vi "Measurement Logic.vi"() -> ()   [LabVIEW 2024, in "Eff And Load Reg_Channel Ganging.lvlib"]
uses:
  Eff And Load Reg_Channel Ganging.lvlib
  Measurement Configuration.ctl
  Measurement Results.ctl
  <vilib>/Plug-In SDKs/Measurements/Measure Call Context/Measure Call Context.lvclass
  <instrlib>/niDCPower/nidcpower.llb/niDCPower Source Mode.ctl
  <instrlib>/niDCPower/nidcpower.llb/niDCPower Output Function.ctl
  <instrlib>/niDCPower/nidcpower.llb/niDCPower Wait For Event - Event.ctl
  shared subVIs/Triggers and Events/NIDCPower_channel_ganging - Configure Digital Edge Source Trigger.vi
  shared subVIs/Triggers and Events/NIDCPower_channel_ganging - Configure Digital Edge Measure Trigger.vi
  <vilib>/Plug-In SDKs/Measurements/Measure Call Context/Accessor/Is Canceled.vi
panel:
  out "measure call context out":refnum<class "Measure Call Context.lvclass">
  in  "measure call context in":refnum<class "Measure Call Context.lvclass">
  out "measurement results":T1
  in  "measurement configuration":T2={"Source master resource name"="", "Source slave resource names"=[], "Load master resource name"="", "Load slave resource names"=[], "Source system configuration"=enum."Parallel", "Source start voltage"=6.0, "Source stop voltage"=14.0, "Source voltage sweep points"=4, "Source voltage level range"=20.0, "Source sense"=1009, "Source limit symmetry"=enum."Asymmetric", "Source current limit range"=25.0, "Source current limit low"=-0.6, "Source current limit high"=25.0, "Source transient response"=1038, "Source voltage gain bandwidth"=2000.0, "Source voltage compensation frequency"=3530.0, "Source voltage pole-zero ratio"=2.0, "Load system configuration"=enum."Parallel", "Load start current"=1.0, "Load stop current"=50.0, "Load current sweep points/points per decade"=10, "Load sweep type"="Logarithmic", "Load current level range"=80.0, "Load sense"=1009, "Load limit symmetry"=enum."Symmetric", "Load voltage limit range"=6.0, "Load voltage limit low"=0.0, "Load voltage limit high"=inf, "Load transient response"=1038, "Load current gain bandwidth"=14000.0, "Load current compensation frequency"=180000.0, "Load current pole-zero ratio"=0.3, "DUT setup time"=1.0, "Source delay"=0.005, "Aperture time"=0.005, "Nominal output voltage"=1.0, "Mode of operation"=enum."Power on the DUT", "Measurement timeout"=0.0} {"Source start voltage" format="%#_6p"; "Load sense" items=["Local"=1008, "Remote"=1009]; "Load transient response" items=["Slow"=1041, "Normal"=1038, "Fast"=1039, "Custom"=1042]; "Source sense" items=["Local"=1008, "Remote"=1009]; "Source transient response" items=["Slow"=1041, "Normal"=1038, "Fast"=1039, "Custom"=1042]; "Load voltage limit high" format="%#_6p"; "Load voltage limit low" format="%#_6p"; "Load voltage limit range" format="%#_6p"; "Source current limit high" format="%#_6p"; "Source current limit low" format="%#_6p"; "Source current limit range" format="%#_6p"; "Source voltage level range" format="%#_6p"}
  out "error out":errorcluster
  in  "error in":errorcluster
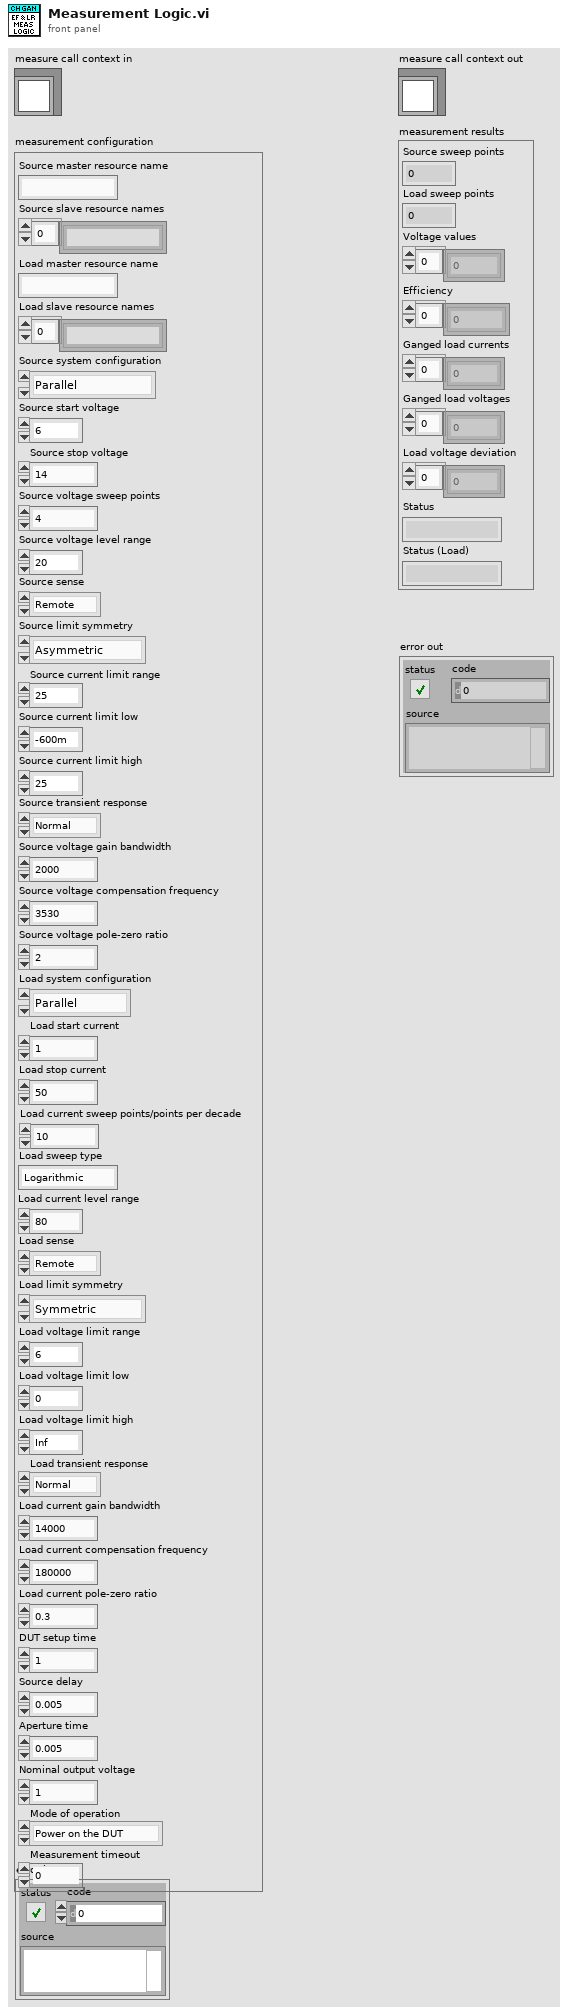
[diagram p1: front panel]
types:
  T1 = typedef "Eff And Load Reg_Channel Ganging.lvlib/Measurement Results.ctl" = cluster{"Source sweep points":i32, "Load sweep points":i32, "Voltage values":dbl[], "Efficiency":dbl[], "Ganged load currents":dbl[], "Ganged load voltages":dbl[], "Load voltage deviation":dbl[], "Status":string, "Status (Load)":string}
  T2 = typedef "Eff And Load Reg_Channel Ganging.lvlib/Measurement Configuration.ctl" = cluster{"Source master resource name":string, "Source slave resource names":string[], "Load master resource name":string, "Load slave resource names":string[], "Source system configuration":enum32{"Series", "Parallel", "Manual"}, "Source start voltage":dbl, "Source stop voltage":dbl, "Source voltage sweep points":i32, "Source voltage level range":dbl, "Source sense":i32, "Source limit symmetry":enum32{"Symmetric", "Asymmetric"}, "Source current limit range":dbl, "Source current limit low":dbl, "Source current limit high":dbl, "Source transient response":i32, "Source voltage gain bandwidth":dbl, "Source voltage compensation frequency":dbl, "Source voltage pole-zero ratio":dbl, "Load system configuration":enum32{"Series", "Parallel", "Manual"}, "Load start current":dbl, "Load stop current":dbl, "Load current sweep points/points per decade":i32, "Load sweep type":string, "Load current level range":dbl, "Load sense":i32, "Load limit symmetry":enum32{"Symmetric", "Asymmetric"}, "Load voltage limit range":dbl, "Load voltage limit low":dbl, "Load voltage limit high":dbl, "Load transient response":i32, "Load current gain bandwidth":dbl, "Load current compensation frequency":dbl, "Load current pole-zero ratio":dbl, "DUT setup time":dbl, "Source delay":dbl, "Aperture time":dbl, "Nominal output voltage":dbl, "Mode of operation":enum32{"Power on the DUT", "Perform measurement", "Power off the DUT"}, "Measurement timeout":dbl}
  T3 = enum32{"Power on the DUT", "Perform measurement", "Power off the DUT"}
  T4 = typedef "niDCPower Output Function.ctl" = i32
  T5 = typedef "niDCPower Source Mode.ctl" = i32
  T6 = typedef "NIDCPower_channel_ganging - ctl - channel def.ctl" = cluster{"resource name":refnum<k15>, "channels":string, "Channel Mode":T7}
  T7 = typedef "NIDCPower_channel_ganging - ctl - channel mode.ctl" = enum32{"Master", "Slave", "Slave - Inverted"}
  T8 = typedef "NIDCPower_channel_ganging - ctl - ganged session.ctl" = cluster{"Ganged Config":T9, "Session List":refnum<k15>[], "Session Mode":T7[], "Channel":string[]}
  T9 = typedef "NIDCPower_channel_ganging - ctl - ganged config.ctl" = enum32{"Series", "Parallel", "Manual"}
  T10 = typedef "niDCPower Wait For Event - Event.ctl" = i32
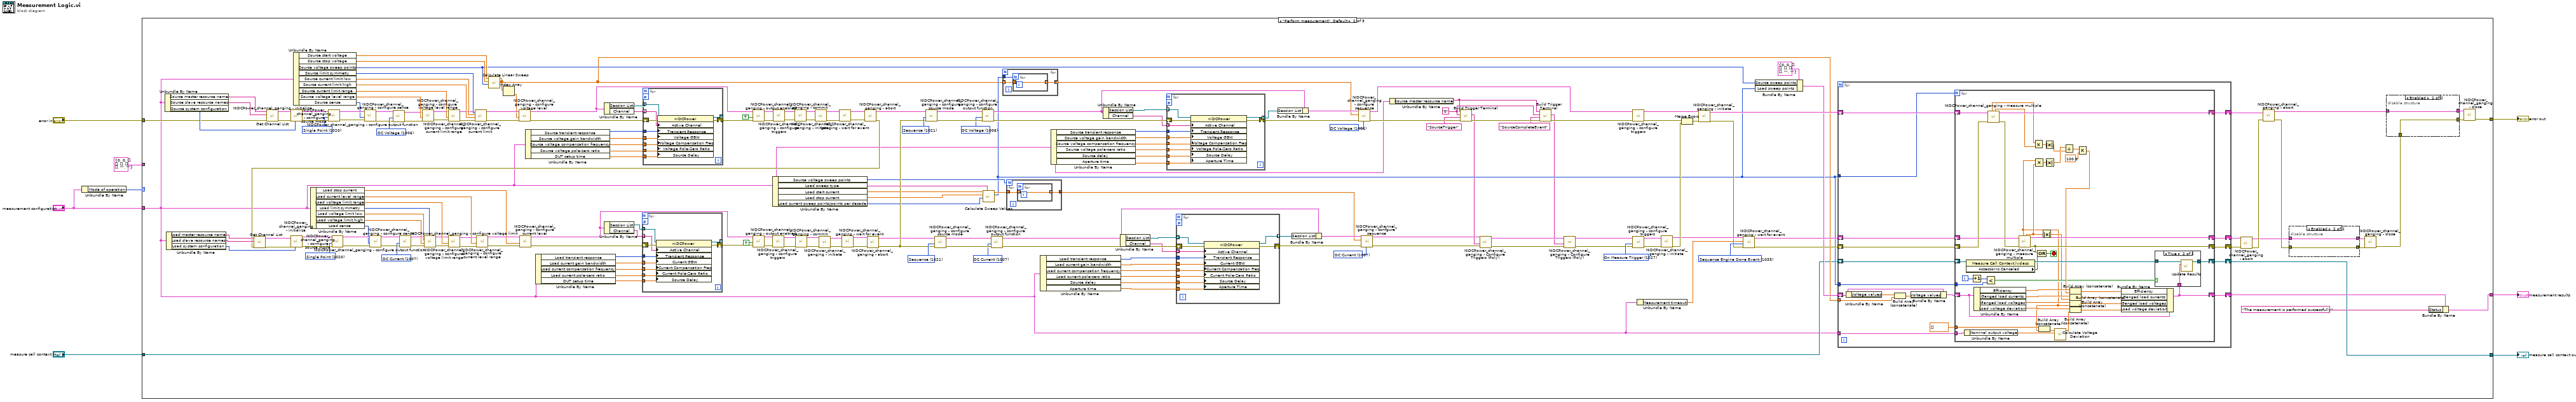
[diagram p0: block diagram]
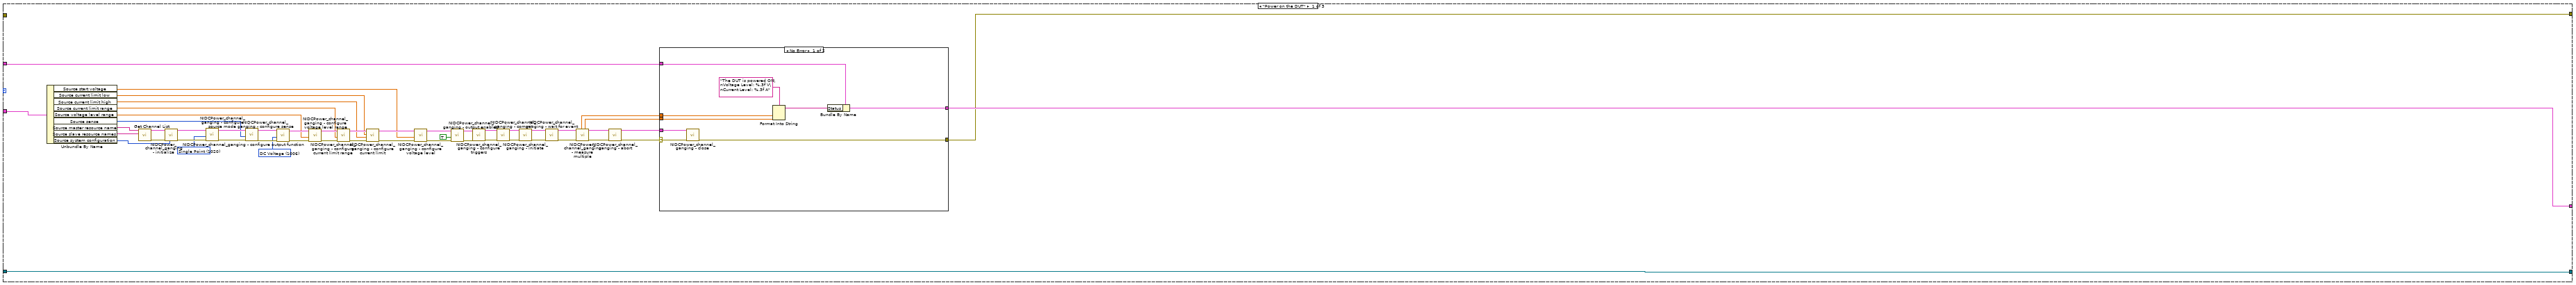
[diagram p2: hidden frame]
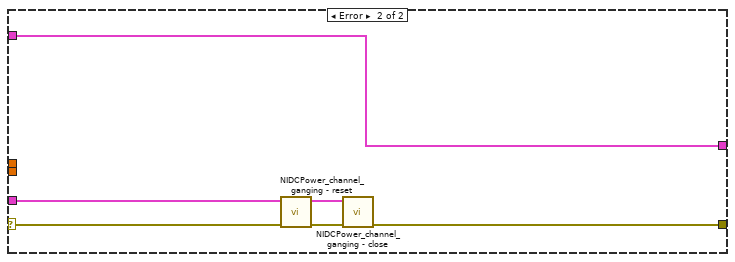
[diagram p3: hidden frame]
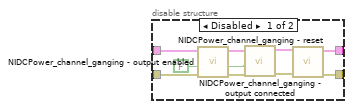
[diagram p4: hidden frame]
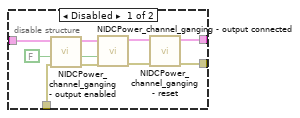
[diagram p5: hidden frame]
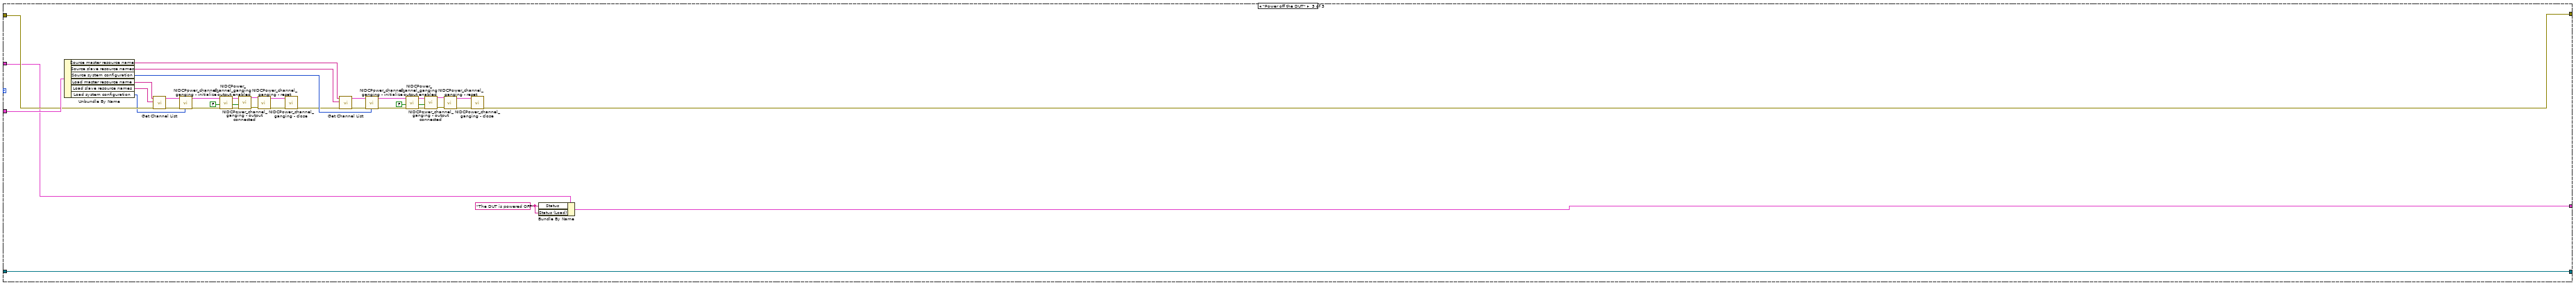
[diagram p7: hidden frame]
diagram:
  n1 = Unbundle By Name("measurement configuration") -> ("Mode of operation"=w3:T3)
  n2 = case shown="\"Perform measurement\", Default" w3 {
    tunnel: [w12 w78 w416] -> w8
    tunnel: [w10 w139 w415] -> w7
    tunnel: [w11 w138 w417] -> w6
    tunnel: "measurement configuration" -> [w14 w76 w448]
    tunnel: "measure call context in" -> [w10 w81 w415]
    tunnel: "error in" -> [_ w80 w442]
    tunnel: T1 {"Source sweep points"=0, "Load sweep points"=0, "Voltage values"=[], "Efficiency"=[], "Ganged load currents"=[], "Ganged load voltages"=[], "Load voltage deviation"=[], "Status"="", "Status (Load)"=""} ("measurement results") -> [w13 _ w418]
    frame "Power on the DUT" {
      w39 = T4 1006 items=["DC Voltage"=1006, "DC Current"=1007, "Pulse Voltage"=1049, "Pulse Current"=1050] ("output function")
      w43 = T5 1020 items=["Single Point"=1020, "Sequence"=1021] ("source mode")
      n3 = Unbundle By Name(w14) -> ("Source start voltage"=w34:dbl, "Source current limit low"=w36:dbl, "Source current limit high"=w35:dbl, "Source current limit range"=w37:dbl, "Source voltage level range"=w38:dbl, "Source sense"=w40:i32, "Source master resource name"=w42:string, "Source slave resource names"=w41:string[], "Source system configuration"=w9:enum32{"Series", "Parallel", "Manual"})
      n4 = call "Get Channel List.vi"("Slave resource names"=w41, "Master resouce name"=w42) -> ("error out"=w44:errorcluster, "Channel List"=w45:T6[])  [unwired: 8 in]
      n5 = call "NIDCPower_channel_ganging - initialize.vi"("Ganged Config"=w9, "error in (no error)"=w44, "Channel List"=w45) -> ("error out"=w58:errorcluster, "Ganged Session Out"=w59:T8)  [unwired: 7 in]
      n6 = call "NIDCPower_channel_ganging - configure source mode.vi"("error in (no error)"=w58, "source mode"=w43, "Ganged Session In"=w59) -> ("error out"=w50:errorcluster, "Ganged Session Out"=w51:T8)  [unwired: 7 in]
      n7 = call "NIDCPower_channel_ganging - configure sense.vi"("error in (no error)"=w50, "sense"=w40, "Ganged Session In"=w51) -> ("error out"=w48:errorcluster, "Ganged Session Out"=w49:T8)  [unwired: 7 in]
      n8 = call "NIDCPower_channel_ganging - configure output function.vi"("error in (no error)"=w48, "output function"=w39, "Ganged Session In"=w49) -> ("error out"=w46:errorcluster, "Ganged Session Out"=w47:T8)  [unwired: 7 in]
      n9 = call "NIDCPower_channel_ganging - configure voltage level range.vi"("error in (no error)"=w46, "voltage level range"=w38, "Ganged Session In"=w47) -> ("error out"=w54:errorcluster, "Ganged Session Out"=w57:T8)  [unwired: 7 in]
      n10 = call "NIDCPower_channel_ganging - configure current limit range.vi"("error in (no error)"=w54, "current limit range"=w37, "Ganged Session In"=w57) -> ("error out"=w53:errorcluster, "Ganged Session Out"=w56:T8)  [unwired: 7 in]
      n11 = call "NIDCPower_channel_ganging - configure current limit.vi"("error in (no error)"=w53, "Current limit/hi"=w35, "Current limit lo"=w36, "Ganged Session In"=w56) -> ("error out"=w52:errorcluster, "Ganged Session Out"=w55:T8)  [unwired: 6 in]
      n12 = call "NIDCPower_channel_ganging - configure voltage level.vi"("error in (no error)"=w52, "voltage level"=w34, "Ganged Session In"=w55) -> ("error out"=w23:errorcluster, "Ganged Session Out"=w24:T8)  [unwired: 7 in]
      n13 = call "NIDCPower_channel_ganging - output enabled.vi"("error in (no error)"=w23, "output enabled"=TRUE, "Ganged Session In"=w24) -> ("error out"=w31:errorcluster, "Ganged Session Out"=w30:T8)  [unwired: 7 in]
      n14 = call "NIDCPower_channel_ganging - configure triggers.vi"("error in (no error)"=w31, "Ganged Session In"=w30) -> ("error out"=w33:errorcluster, "Ganged Session Out"=w32:T8)  [unwired: 8 in]
      n15 = call "NIDCPower_channel_ganging - commit.vi"("error in (no error)"=w33, "Ganged Session In"=w32) -> ("error out"=w28:errorcluster, "Ganged Session Out"=w29:T8)  [unwired: 8 in]
      n16 = call "NIDCPower_channel_ganging - initiate.vi"("error in (no error)"=w28, "Ganged Session In"=w29) -> ("error out"=w26:errorcluster, "Ganged Session Out"=w27:T8)  [unwired: 8 in]
      n17 = call "NIDCPower_channel_ganging - wait for event.vi"("error in (no error)"=w26, "Ganged Session in"=w27) -> ("error out"=w21:errorcluster, "Ganged Session Out"=w22:T8)  [unwired: 8 in]
      n18 = call "NIDCPower_channel_ganging - measure multiple.vi"("error in (no error)"=w21, "Ganged Session In"=w22) -> ("error out"=w19:errorcluster, "Ganged Session Out"=w20:T8, "ganged current measurement"=w15:dbl, "ganged voltage measurement"=w16:dbl)  [unwired: 2 in, 4 out]
      n19 = call "NIDCPower_channel_ganging - abort.vi"("error in (no error)"=w19, "Ganged Session In"=w20) -> ("error out"=w18:errorcluster, "Ganged Session Out"=w17:T8)  [unwired: 8 in]
      n20 = case shown="No Error" w18 {
        selector: w18 -> [w67 w72]
        tunnel: w17 -> [w68 w74]
        tunnel: w16 -> [w66 _]
        tunnel: w15 -> [w65 _]
        tunnel: w13 -> [w63 w70]
        tunnel: [w61 w69] -> w11
        tunnel: [w60 w70] -> w12
        frame No Error {
          n21 = call "NIDCPower_channel_ganging - close.vi"("error in (no error)"=w67, "Ganged Session In"=w68) -> ("error out"=w61:errorcluster)  [unwired: 9 in]
          n22 = Format Into String(format string="The DUT is powered ON\nVoltage Level: %.3f V\nCurrent Level: %.3f A", w66, w65) -> (resulting string=w62:string)  [unwired: 2 in, 1 out]
          n23 = Bundle By Name(cluster=w63, "Status"=w62) -> (w60:T1)
        }
        frame Error {
          n24 = call "NIDCPower_channel_ganging - reset.vi"("error in (no error)"=w72, "Ganged Session In"=w74) -> ("error out"=w71:errorcluster, "Ganged Session Out"=w73:T8)  [unwired: 8 in]
          n25 = call "NIDCPower_channel_ganging - close.vi"("error in (no error)"=w71, "Ganged Session In"=w73) -> ("error out"=w69:errorcluster)  [unwired: 9 in]
        }
      }
    }
    frame "Perform measurement", Default {
      w103 = T4 1007 items=["DC Voltage"=1006, "DC Current"=1007, "Pulse Voltage"=1049, "Pulse Current"=1050] ("output function")
      w104 = T4 1006 items=["DC Voltage"=1006, "DC Current"=1007, "Pulse Voltage"=1049, "Pulse Current"=1050] ("output function")
      w133 = "0" ("Channel Name")
      w178 = 1027 items=["Automatically after Source Complete"=1025, "On Demand"=1026, "On Measure Trigger"=1027] ("Measure When")
      w175 = T4 1006 items=["DC Voltage"=1006, "DC Current"=1007, "Pulse Voltage"=1049, "Pulse Current"=1050] ("output function")
      w180 = T5 1021 items=["Single Point"=1020, "Sequence"=1021] ("source mode")
      w181 = T5 1021 items=["Single Point"=1020, "Sequence"=1021] ("source mode")
      w112 = T4 1007 items=["DC Voltage"=1006, "DC Current"=1007, "Pulse Voltage"=1049, "Pulse Current"=1050] ("output function")
      w228 = T10 1033 items=["Source Complete Event"=1030, "Measure Complete Event"=1031, "Sequence Iteration Complete Event"=1032, "Sequence Engine Done Event"=1033, "Pulse Complete Event"=1051, "Ready For Pulse Trigger Event"=1052] ("event")
      w229 = T4 1007 items=["DC Voltage"=1006, "DC Current"=1007, "Pulse Voltage"=1049, "Pulse Current"=1050] ("output function")
      w242 = T4 1006 items=["DC Voltage"=1006, "DC Current"=1007, "Pulse Voltage"=1049, "Pulse Current"=1050] ("output function")
      w274 = T5 1020 items=["Single Point"=1020, "Sequence"=1021] ("source mode")
      w275 = T5 1020 items=["Single Point"=1020, "Sequence"=1021] ("source mode")
      n26 = Unbundle By Name(w76) -> ("Source master resource name"=w124:string, "Source slave resource names"=w123:string[], "Source system configuration"=w253:enum32{"Series", "Parallel", "Manual"})
      n27 = Unbundle By Name(w76) -> ("Load master resource name"=w120:string, "Load slave resource names"=w119:string[], "Load system configuration"=w252:enum32{"Series", "Parallel", "Manual"})
      n28 = call "Get Channel List.vi"("error in (no error)"=w80, "Slave resource names"=w123, "Master resouce name"=w124) -> ("error out"=w125:errorcluster, "Channel List"=w126:T6[])  [unwired: 7 in]
      n29 = call "NIDCPower_channel_ganging - initialize.vi"("Ganged Config"=w253, "error in (no error)"=w125, "Channel List"=w126) -> ("error out"=w276:errorcluster, "Ganged Session Out"=w277:T8)  [unwired: 7 in]
      n30 = Unbundle By Name(w76) -> ("Source start voltage"=w155:dbl, "Source stop voltage"=w154:dbl, "Source voltage sweep points"=w142:i32, "Source limit symmetry"=w259:enum32{"Symmetric", "Asymmetric"}, "Source current limit low"=w260:dbl, "Source current limit high"=w261:dbl, "Source current limit range"=w262:dbl, "Source voltage level range"=w263:dbl, "Source sense"=w130:i32)
      n31 = Unbundle By Name(w76) -> ("Load stop current"=w144:dbl, "Load current level range"=w254:dbl, "Load voltage limit range"=w255:dbl, "Load limit symmetry"=w258:enum32{"Symmetric", "Asymmetric"}, "Load voltage limit low"=w257:dbl, "Load voltage limit high"=w256:dbl, "Load sense"=w131:i32)
      n32 = call "NIDCPower_channel_ganging - configure source mode.vi"("error in (no error)"=w276, "source mode"=w275, "Ganged Session In"=w277) -> ("error out"=w225:errorcluster, "Ganged Session Out"=w226:T8)  [unwired: 7 in]
      n33 = call "NIDCPower_channel_ganging - configure sense.vi"("error in (no error)"=w225, "sense"=w130, "Ganged Session In"=w226) -> ("error out"=w223:errorcluster, "Ganged Session Out"=w224:T8)  [unwired: 7 in]
      n34 = call "NIDCPower_channel_ganging - configure output function.vi"("error in (no error)"=w223, "output function"=w242, "Ganged Session In"=w224) -> ("error out"=w221:errorcluster, "Ganged Session Out"=w222:T8)  [unwired: 7 in]
      n35 = call "NIDCPower_channel_ganging - configure voltage level range.vi"("error in (no error)"=w221, "voltage level range"=w263, "Ganged Session In"=w222) -> ("error out"=w238:errorcluster, "Ganged Session Out"=w241:T8)  [unwired: 7 in]
      n36 = call "NIDCPower_channel_ganging - configure current limit range.vi"("error in (no error)"=w238, "current limit range"=w262, "Ganged Session In"=w241) -> ("error out"=w237:errorcluster, "Ganged Session Out"=w240:T8)  [unwired: 7 in]
      n37 = call "NIDCPower_channel_ganging - configure current limit.vi"("Limit Symmetry"=w259, "error in (no error)"=w237, "Current limit/hi"=w261, "Current limit lo"=w260, "Ganged Session In"=w240) -> ("error out"=w236:errorcluster, "Ganged Session Out"=w239:T8)  [unwired: 5 in]
      n38 = call "Calculate Linear Sweep.vi"("Points"=w142, "Stop level"=w154, "Start level"=w155) -> ("Values"=w132:dbl[])  [unwired: 8 in]
      n39 = Index Array(array=w132) -> (element=w156:dbl)  [unwired: 1 in]
      n40 = call "NIDCPower_channel_ganging - configure voltage level.vi"("error in (no error)"=w236, "voltage level"=w156, "Ganged Session In"=w239) -> ("error out"=w196:errorcluster, "Ganged Session Out"=w190:T8)  [unwired: 7 in]
      n41 = Unbundle By Name(w76) -> ("Source transient response"=w97:i32, "Source voltage gain bandwidth"=w93:dbl, "Source voltage compensation frequency"=w92:dbl, "Source voltage pole-zero ratio"=w91:dbl, "DUT setup time"=w94:dbl)
      n42 = Unbundle By Name(w76) -> ("Load transient response"=w96:i32, "Load current gain bandwidth"=w90:dbl, "Load current compensation frequency"=w89:dbl, "Load current pole-zero ratio"=w88:dbl, "DUT setup time"=w95:dbl)
      n43 = Unbundle By Name(w190) -> ("Session List"=w194:refnum<k15>[], "Channel"=w193:string[])
      n44 = for {
        tunnel: [w337] -> _ mode=indexing
        shift-right: [w335] -> w195
        shift-left: w196 -> [w336]
        workers-P: _ -> [_]
        tunnel: w194 -> [w334] mode=indexing
        tunnel: w193 -> [w333] mode=indexing
        tunnel: w97 -> [w332]
        tunnel: w94 -> [w331]
        tunnel: w93 -> [w330]
        tunnel: w92 -> [w329]
        tunnel: w91 -> [w328]
        n45 = property class="niDCPower"(reference=w334, error in=w336, "Active Channel"=w333, "Transient Response"=w332, "Voltage GBW"=w330, "Voltage Compensation Freq"=w329, "Voltage Pole-Zero Ratio"=w328, "Source Delay"=w331) -> (reference out=w337:refnum<k15>, error out=w335:errorcluster)
      }
      n46 = call "NIDCPower_channel_ganging - output enabled.vi"("error in (no error)"=w195, "output enabled"=TRUE, "Ganged Session In"=w190) -> ("error out"=w199:errorcluster, "Ganged Session Out"=w200:T8)  [unwired: 7 in]
      n47 = Unbundle By Name(w76) -> ("Source voltage sweep points"=w145:i32, "Load sweep type"=w129:string, "Load start current"=w153:dbl, "Load stop current"=w152:dbl, "Load current sweep points/points per decade"=w151:i32)
      n48 = call "NIDCPower_channel_ganging - configure triggers.vi"("error in (no error)"=w199, "Ganged Session In"=w200) -> ("error out"=w197:errorcluster, "Ganged Session Out"=w198:T8)  [unwired: 8 in]
      n49 = call "NIDCPower_channel_ganging - commit.vi"("error in (no error)"=w197, "Ganged Session In"=w198) -> ("error out"=w206:errorcluster, "Ganged Session Out"=w205:T8)  [unwired: 8 in]
      n50 = call "NIDCPower_channel_ganging - initiate.vi"("error in (no error)"=w206, "Ganged Session In"=w205) -> ("error out"=w208:errorcluster, "Ganged Session Out"=w207:T8)  [unwired: 8 in]
      n51 = call "NIDCPower_channel_ganging - wait for event.vi"("error in (no error)"=w208, "Ganged Session in"=w207) -> ("error out"=w210:errorcluster, "Ganged Session Out"=w209:T8)  [unwired: 8 in]
      n52 = call "NIDCPower_channel_ganging - abort.vi"("error in (no error)"=w210, "Ganged Session In"=w209) -> ("error out"=w118:errorcluster, "Ganged Session Out"=w179:T8)  [unwired: 8 in]
      n53 = call "Get Channel List.vi"("error in (no error)"=w118, "Slave resource names"=w119, "Master resouce name"=w120) -> ("error out"=w122:errorcluster, "Channel List"=w121:T6[])  [unwired: 7 in]
      n54 = call "NIDCPower_channel_ganging - initialize.vi"("Ganged Config"=w252, "error in (no error)"=w122, "Channel List"=w121) -> ("error out"=w273:errorcluster, "Ganged Session Out"=w272:T8)  [unwired: 7 in]
      n55 = call "NIDCPower_channel_ganging - configure source mode.vi"("error in (no error)"=w273, "source mode"=w274, "Ganged Session In"=w272) -> ("error out"=w219:errorcluster, "Ganged Session Out"=w220:T8)  [unwired: 7 in]
      n56 = call "NIDCPower_channel_ganging - configure sense.vi"("error in (no error)"=w219, "sense"=w131, "Ganged Session In"=w220) -> ("error out"=w217:errorcluster, "Ganged Session Out"=w218:T8)  [unwired: 7 in]
      n57 = call "NIDCPower_channel_ganging - configure output function.vi"("error in (no error)"=w217, "output function"=w229, "Ganged Session In"=w218) -> ("error out"=w270:errorcluster, "Ganged Session Out"=w271:T8)  [unwired: 7 in]
      n58 = call "NIDCPower_channel_ganging - configure voltage limit.vi"("Limit Symmetry"=w258, "error in (no error)"=w270, "voltage limit/hi"=w256, "voltage limit lo"=w257, "Ganged Session In"=w271) -> ("error out"=w234:errorcluster, "Ganged Session Out"=w235:T8)  [unwired: 5 in]
      n59 = call "NIDCPower_channel_ganging - configure voltage limit range.vi"("error in (no error)"=w234, "voltage level range"=w255, "Ganged Session In"=w235) -> ("error out"=w232:errorcluster, "Ganged Session Out"=w233:T8)  [unwired: 7 in]
      n60 = call "NIDCPower_channel_ganging - configure current level range.vi"("error in (no error)"=w232, "current level range"=w254, "Ganged Session In"=w233) -> ("error out"=w230:errorcluster, "Ganged Session Out"=w231:T8)  [unwired: 7 in]
      n61 = call "NIDCPower_channel_ganging - configure current level.vi"("error in (no error)"=w230, "current level"=w144, "Ganged Session In"=w231) -> ("error out"=w192:errorcluster, "Ganged Session Out"=w189:T8)  [unwired: 7 in]
      n62 = Unbundle By Name(w189) -> ("Session List"=w188:refnum<k15>[], "Channel"=w187:string[])
      n63 = for {
        tunnel: [w327] -> _ mode=indexing
        shift-right: [w325] -> w191
        shift-left: w192 -> [w326]
        workers-P: _ -> [_]
        tunnel: w188 -> [w324] mode=indexing
        tunnel: w187 -> [w323] mode=indexing
        tunnel: w96 -> [w322]
        tunnel: w95 -> [w321]
        tunnel: w90 -> [w320]
        tunnel: w89 -> [w319]
        tunnel: w88 -> [w318]
        n64 = property class="niDCPower"(reference=w324, error in=w326, "Active Channel"=w323, "Transient Response"=w322, "Current GBW"=w320, "Current Compensation Freq"=w319, "Current Pole-Zero Ratio"=w318, "Source Delay"=w321) -> (reference out=w327:refnum<k15>, error out=w325:errorcluster)
      }
      n65 = call "NIDCPower_channel_ganging - output enabled.vi"("error in (no error)"=w191, "output enabled"=TRUE, "Ganged Session In"=w189) -> ("error out"=w203:errorcluster, "Ganged Session Out"=w204:T8)  [unwired: 7 in]
      n66 = call "NIDCPower_channel_ganging - configure triggers.vi"("error in (no error)"=w203, "Ganged Session In"=w204) -> ("error out"=w201:errorcluster, "Ganged Session Out"=w202:T8)  [unwired: 8 in]
      n67 = call "NIDCPower_channel_ganging - commit.vi"("error in (no error)"=w201, "Ganged Session In"=w202) -> ("error out"=w215:errorcluster, "Ganged Session Out"=w216:T8)  [unwired: 8 in]
      n68 = call "NIDCPower_channel_ganging - initiate.vi"("error in (no error)"=w215, "Ganged Session In"=w216) -> ("error out"=w213:errorcluster, "Ganged Session Out"=w214:T8)  [unwired: 8 in]
      n69 = call "NIDCPower_channel_ganging - wait for event.vi"("error in (no error)"=w213, "Ganged Session in"=w214) -> ("error out"=w211:errorcluster, "Ganged Session Out"=w212:T8)  [unwired: 8 in]
      n70 = call "NIDCPower_channel_ganging - abort.vi"("error in (no error)"=w211, "Ganged Session In"=w212) -> ("error out"=w157:errorcluster, "Ganged Session Out"=w182:T8)  [unwired: 8 in]
      n71 = call "NIDCPower_channel_ganging - configure source mode.vi"("error in (no error)"=w157, "source mode"=w180, "Ganged Session In"=w179) -> ("error out"=w183:errorcluster, "Ganged Session Out"=w184:T8)  [unwired: 7 in]
      n72 = call "NIDCPower_channel_ganging - configure source mode.vi"("error in (no error)"=w157, "source mode"=w181, "Ganged Session In"=w182) -> ("error out"=w186:errorcluster, "Ganged Session Out"=w185:T8)  [unwired: 7 in]
      n73 = call "NIDCPower_channel_ganging - configure output function.vi"("error in (no error)"=w183, "output function"=w175, "Ganged Session In"=w184) -> ("error out"=w176:errorcluster, "Ganged Session Out"=w177:T8)  [unwired: 7 in]
      n74 = call "Calculate Sweep Values.vi"("Sweep type"=w129, "Points"=w151, "Stop level"=w152, "Start level"=w153) -> ("Sweep points"=w141:i32, "Sweep values"=w150:dbl[])  [unwired: 5 in, 1 out]
      n75 = call "NIDCPower_channel_ganging - configure output function.vi"("error in (no error)"=w186, "output function"=w112, "Ganged Session In"=w185) -> ("error out"=w162:errorcluster, "Ganged Session Out"=w163:T8)  [unwired: 7 in]
      n76 = for {
        tunnel: w132 -> [w302] mode=indexing
        tunnel: [w301] -> w109 mode=concatenating
        tunnel: w141 -> [w300]
        n77 = for {
          N: w300 -> [_]
          tunnel: w302 -> [w303]
          tunnel: [w303] -> w301 mode=indexing
        }
      }
      n78 = for {
        N: w145 -> [_]
        tunnel: w150 -> [w305]
        tunnel: [w304] -> w113 mode=concatenating
        n79 = for {
          tunnel: w305 -> [w306] mode=indexing
          tunnel: [w306] -> w304 mode=indexing
        }
      }
      n80 = Unbundle By Name(w76) -> ("Load transient response"=w102:i32, "Load current gain bandwidth"=w84:dbl, "Load current compensation frequency"=w83:dbl, "Load current pole-zero ratio"=w82:dbl, "Source delay"=w101:dbl, "Aperture time"=w100:dbl)
      n81 = Unbundle By Name(w76) -> ("Source transient response"=w105:i32, "Source voltage gain bandwidth"=w87:dbl, "Source voltage compensation frequency"=w86:dbl, "Source voltage pole-zero ratio"=w85:dbl, "Source delay"=w99:dbl, "Aperture time"=w98:dbl)
      n82 = Unbundle By Name(w177) -> ("Session List"=w267:refnum<k15>[], "Channel"=w161:string[])
      n83 = Unbundle By Name(w163) -> ("Session List"=w160:refnum<k15>[], "Channel"=w159:string[])
      n84 = for {
        tunnel: [w348] -> w266 mode=indexing
        shift-right: [w346] -> w108
        shift-left: w176 -> [w347]
        workers-P: _ -> [_]
        tunnel: w267 -> [w345] mode=indexing
        tunnel: w161 -> [w344] mode=indexing
        tunnel: w105 -> [w343]
        tunnel: w99 -> [w342]
        tunnel: w98 -> [w341]
        tunnel: w87 -> [w340]
        tunnel: w86 -> [w339]
        tunnel: w85 -> [w338]
        n85 = property class="niDCPower"(reference=w345, error in=w347, "Active Channel"=w344, "Transient Response"=w343, "Voltage GBW"=w340, "Voltage Compensation Freq"=w339, "Voltage Pole-Zero Ratio"=w338, "Source Delay"=w342, "Aperture Time"=w341) -> (reference out=w348:refnum<k15>, error out=w346:errorcluster)
      }
      n86 = for {
        tunnel: [w317] -> w158 mode=indexing
        shift-right: [w315] -> w116
        shift-left: w162 -> [w316]
        workers-P: _ -> [_]
        tunnel: w160 -> [w314] mode=indexing
        tunnel: w159 -> [w313] mode=indexing
        tunnel: w102 -> [w312]
        tunnel: w101 -> [w311]
        tunnel: w100 -> [w310]
        tunnel: w84 -> [w309]
        tunnel: w83 -> [w308]
        tunnel: w82 -> [w307]
        n87 = property class="niDCPower"(reference=w314, error in=w316, "Active Channel"=w313, "Transient Response"=w312, "Current GBW"=w309, "Current Compensation Freq"=w308, "Current Pole-Zero Ratio"=w307, "Source Delay"=w311, "Aperture Time"=w310) -> (reference out=w317:refnum<k15>, error out=w315:errorcluster)
      }
      n88 = Bundle By Name(cluster=w177, "Session List"=w266) -> (w111:T8)
      n89 = Bundle By Name(cluster=w163, "Session List"=w158) -> (w117:T8)
      n90 = call "NIDCPower_channel_ganging - confgure sequence.vi"("output function"=w104, "error in (no error)"=w108, "Values"=w109, "Ganged Session In"=w111) -> ("error out"=w107:errorcluster, "Ganged Session Out"=w110:T8)  [unwired: 6 in]
      n91 = call "NIDCPower_channel_ganging - confgure sequence.vi"("output function"=w103, "error in (no error)"=w116, "Values"=w113, "Ganged Session In"=w117) -> ("error out"=w114:errorcluster, "Ganged Session Out"=w115:T8)  [unwired: 6 in]
      n92 = Unbundle By Name(w76) -> ("Source master resource name"=w106:string)
      n93 = call "Build Trigger Terminal.vi"("error in (no error)"=w107, "Trigger/Event Name"="SourceTrigger", "Channel Name"=w133, "Resource Name"=w106) -> ("error out"=w149:errorcluster, "Terminal Name"=w128:string)  [unwired: 6 in]
      n94 = call-poly "NIDCPower_channel_ganging - Configure Triggers (Poly).vi"("error in (no error)"=w114, "output terminal"=w128, "Ganged Session in"=w115) -> ("error out"=w134:errorcluster, "Ganged Session out"=w135:T8)  [unwired: 7 in]
      n95 = call "Build Trigger Terminal.vi"("error in (no error)"=w149, "Trigger/Event Name"="SourceCompleteEvent", "Channel Name"=w133, "Resource Name"=w106) -> ("error out"=w148:errorcluster, "Terminal Name"=w127:string)  [unwired: 6 in]
      n96 = call-poly "NIDCPower_channel_ganging - Configure Triggers (Poly).vi"("error in (no error)"=w134, "output terminal"=w127, "Ganged Session in"=w135) -> ("error out"=w136:errorcluster, "Ganged Session out"=w137:T8)  [unwired: 7 in]
      n97 = call "NIDCPower_channel_ganging - configure triggers.vi"("error in (no error)"=w148, "Ganged Session In"=w110) -> ("error out"=w244:errorcluster, "Ganged Session Out"=w245:T8)  [unwired: 8 in]
      n98 = call "NIDCPower_channel_ganging - configure triggers.vi"("error in (no error)"=w136, "Measure When"=w178, "Ganged Session In"=w137) -> ("error out"=w264:errorcluster, "Ganged Session Out"=w265:T8)  [unwired: 7 in]
      n99 = Unbundle By Name(w76) -> ("Measurement timeout"=w75:dbl)
      n100 = call "NIDCPower_channel_ganging - initiate.vi"("error in (no error)"=w264, "Ganged Session In"=w265) -> ("error out"=w243:errorcluster, "Ganged Session Out"=w227:T8)  [unwired: 8 in]
      n101 = Merge Errors(w244, w243) -> (w246:errorcluster)
      n102 = call "NIDCPower_channel_ganging - initiate.vi"("error in (no error)"=w246, "Ganged Session In"=w245) -> ("error out"=w174:errorcluster, "Ganged Session Out"=w165:T8)  [unwired: 8 in]
      n103 = call "NIDCPower_channel_ganging - wait for event.vi"("error in (no error)"=w174, "event"=w228, "timeout (10.0)"=w75, "Ganged Session in"=w227) -> ("error out"=w169:errorcluster, "Ganged Session Out"=w167:T8)  [unwired: 6 in]
      n104 = Bundle By Name(cluster=T1 {"Source sweep points"=0, "Load sweep points"=0, "Voltage values"=[], "Efficiency"=[], "Ganged load currents"=[], "Ganged load voltages"=[], "Load voltage deviation"=[], "Status"="", "Status (Load)"=""} ("Measurement Results"), "Source sweep points"=w142, "Load sweep points"=w141) -> (w143:T1)
      n105 = for {
        shift-right: [w365] -> w168
        shift-left: w169 -> [w366]
        shift-right: [w363] -> w166
        shift-left: w167 -> [w364]
        shift-right: [w361] -> w164
        shift-left: w165 -> [w362]
        tunnel: w141 -> [w360]
        shift-right: [w358] -> w139
        shift-left: w81 -> [w359]
        shift-right: [w357] -> w79
        shift-left: w143 -> [w352]
        tunnel: w141 -> [w356]
        tunnel: w132 -> [w351] mode=indexing
        tunnel: w76 -> [w350]
        n106 = Unbundle By Name(w352) -> ("Voltage values"=w355:dbl[])
        n107 = Build Array (concatenate)(w355, w351) -> (w354:dbl[])
        n108 = Bundle By Name(cluster=w352, "Voltage values"=w354) -> (w353:T1)
        n109 = for {
          N: w360 -> [_]
          shift-right: [w398] -> w365
          shift-left: w366 -> [w407]
          shift-right: [w408] -> w363
          shift-left: w364 -> [w409]
          shift-right: [w404] -> w361
          shift-left: w362 -> [w405]
          shift-right: [w401] -> w358
          shift-left: w359 -> [w403]
          shift-right: [w389] -> w357
          shift-left: w353 -> [w370]
          tunnel: w356 -> [w385]
          tunnel: w350 -> [w368]
          tunnel: dbl[] [] ("Efficiency") -> [w373]
          i -> [w386]
          stop <- w400 stop-if-true
          n110 = Unbundle By Name(w368) -> ("Nominal output voltage"=w374:dbl)
          n111 = property class="Measure Call Context.lvclass"(reference=w403) -> (reference out=w402:refnum<class "Measure Call Context.lvclass">, "Accessor:Is Canceled"=w399:bool)  [unwired: 1 in, 1 out]
          n112 = Increment(x=w386) -> (x+1=w387:i32)
          n113 = Unbundle By Name(w370) -> ("Efficiency"=w397:dbl[], "Ganged load currents"=w392:dbl[], "Ganged load voltages"=w375:dbl[], "Load voltage deviation"=w378:dbl[])
          n114 = Less?(x=w387, y=w385) -> (x < y?=w384:bool)
          n115 = call "NIDCPower_channel_ganging - measure multiple.vi"("error in (no error)"=w407, "Ganged Session In"=w405) -> ("error out"=w406:errorcluster, "Ganged Session Out"=w404:T8, "ganged current measurement"=w382:dbl, "ganged voltage measurement"=w381:dbl)  [unwired: 2 in, 4 out]
          n116 = call "NIDCPower_channel_ganging - measure multiple.vi"("error in (no error)"=w406, "Ganged Session In"=w409) -> ("error out"=w398:errorcluster, "Ganged Session Out"=w408:T8, "ganged current measurement"=w383:dbl, "ganged voltage measurement"=w372:dbl)  [unwired: 2 in, 4 out]
          n117 = Multiply(x=w381, y=w382) -> (x*y=w394:dbl)
          n118 = Multiply(x=w372, y=w383) -> (x*y=w393:dbl)
          n119 = Compound Arithmetic op=OR(w398, w399) -> (w400:bool)
          n120 = Build Array (concatenate)(w373, w372) -> (w371:dbl[])
          n121 = Absolute Value(x=w383) -> (abs(x)=w367:dbl)
          n122 = Absolute Value(x=w394) -> (abs(x)=w380:dbl)
          n123 = Absolute Value(x=w393) -> (abs(x)=w379:dbl)
          n124 = call "Calculate Voltage Deviation.vi"("Nominal output voltage"=w374, "Voltage measurements"=w371) -> ("Load voltage deviation"=w377:dbl[])  [unwired: 9 in]
          n125 = Divide(x=w379, y=w380) -> (x/y=w396:dbl)
          n126 = Build Array (concatenate)(w392, w367) -> (w390:dbl[])
          n127 = Build Array (concatenate)(w375, w372) -> (w369:dbl[])
          n128 = Build Array (concatenate)(w378, w377) -> (w376:dbl[])
          n129 = Multiply(x=w396, y=100.0) -> (x*y=w388:dbl)
          n130 = Build Array (concatenate)(w397, w388) -> (w391:dbl[])
          n131 = Bundle By Name(cluster=w370, "Efficiency"=w391, "Ganged load currents"=w390, "Ganged load voltages"=w369, "Load voltage deviation"=w376) -> (w389:T1)
          n132 = case shown="True" w384 {
            tunnel: w389 -> [_ w413]
            tunnel: w402 -> [w410 w412]
            tunnel: [w410 w411] -> w401
            frame False {
            }
            frame True {
              n133 = call <vilib>:"Update Results.vi"("measurement results"=w413, "measure call context in"=w412) -> ("measure call context out"=w411:refnum<class "Measure Call Context.lvclass">)  [unwired: 8 in, 1 out]
            }
          }
        }
      }
      n134 = call "NIDCPower_channel_ganging - abort.vi"("error in (no error)"=w168, "Ganged Session In"=w166) -> ("error out"=w251:errorcluster, "Ganged Session Out"=w249:T8)  [unwired: 8 in]
      n135 = call "NIDCPower_channel_ganging - abort.vi"("error in (no error)"=w251, "Ganged Session In"=w164) -> ("error out"=w250:errorcluster, "Ganged Session Out"=w247:T8)  [unwired: 8 in]
      n136 = disable-structure shown="Enabled" {
        disable-tunnel: w250 -> [w286 w287]
        disable-tunnel: w249 -> [w283 w288]
        disable-tunnel: [w279 w288] -> w173
        disable-tunnel: [w278 w287] -> w172
        frame Disabled {
          w282 = FALSE ("output enabled")
          n137 = call "NIDCPower_channel_ganging - output enabled.vi"("error in (no error)"=w286, "output enabled"=w282, "Ganged Session In"=w283) -> ("error out"=w284:errorcluster, "Ganged Session Out"=w285:T8)  [unwired: 7 in]
          n138 = call "NIDCPower_channel_ganging - output connected.vi"("error in (no error)"=w284, "output enabled"=w282, "Ganged Session In"=w285) -> ("error out"=w281:errorcluster, "Ganged Session Out"=w280:T8)  [unwired: 7 in]
          n139 = call "NIDCPower_channel_ganging - reset.vi"("error in (no error)"=w281, "Ganged Session In"=w280) -> ("error out"=w278:errorcluster, "Ganged Session Out"=w279:T8)  [unwired: 8 in]
        }
        frame Enabled {
        }
      }
      n140 = call "NIDCPower_channel_ganging - close.vi"("error in (no error)"=w172, "Ganged Session In"=w173) -> ("error out"=w248:errorcluster)  [unwired: 9 in]
      n141 = disable-structure shown="Enabled" {
        disable-tunnel: w248 -> [w295 w298]
        disable-tunnel: w247 -> [w294 w299]
        disable-tunnel: [w290 w299] -> w171
        disable-tunnel: [w289 w298] -> w170
        frame Disabled {
          w293 = FALSE ("output enabled")
          n142 = call "NIDCPower_channel_ganging - output enabled.vi"("error in (no error)"=w295, "output enabled"=w293, "Ganged Session In"=w294) -> ("error out"=w297:errorcluster, "Ganged Session Out"=w296:T8)  [unwired: 7 in]
          n143 = call "NIDCPower_channel_ganging - output connected.vi"("error in (no error)"=w297, "output enabled"=w293, "Ganged Session In"=w296) -> ("error out"=w291:errorcluster, "Ganged Session Out"=w292:T8)  [unwired: 7 in]
          n144 = call "NIDCPower_channel_ganging - reset.vi"("error in (no error)"=w291, "Ganged Session In"=w292) -> ("error out"=w289:errorcluster, "Ganged Session Out"=w290:T8)  [unwired: 8 in]
        }
        frame Enabled {
        }
      }
      n145 = Bundle By Name(cluster=w79, "Status"="The measurement is performed successfully") -> (w78:T1)
      n146 = call "NIDCPower_channel_ganging - close.vi"("error in (no error)"=w170, "Ganged Session In"=w171) -> ("error out"=w138:errorcluster)  [unwired: 9 in]
    }
    frame "Power off the DUT" {
      w414 = "The DUT is powered OFF"
      w426 = FALSE ("output enabled")
      w443 = FALSE ("output enabled")
      n147 = Unbundle By Name(w448) -> ("Source master resource name"=w420:string, "Source slave resource names"=w419:string[], "Source system configuration"=w449:enum32{"Series", "Parallel", "Manual"}, "Load master resource name"=w441:string, "Load slave resource names"=w440:string[], "Load system configuration"=w437:enum32{"Series", "Parallel", "Manual"})
      n148 = call "Get Channel List.vi"("error in (no error)"=w442, "Slave resource names"=w440, "Master resouce name"=w441) -> ("error out"=w438:errorcluster, "Channel List"=w439:T6[])  [unwired: 7 in]
      n149 = call "NIDCPower_channel_ganging - initialize.vi"("Ganged Config"=w437, "error in (no error)"=w438, "Channel List"=w439) -> ("error out"=w436:errorcluster, "Ganged Session Out"=w435:T8)  [unwired: 7 in]
      n150 = call "NIDCPower_channel_ganging - output enabled.vi"("error in (no error)"=w436, "output enabled"=w443, "Ganged Session In"=w435) -> ("error out"=w445:errorcluster, "Ganged Session Out"=w444:T8)  [unwired: 7 in]
      n151 = call "NIDCPower_channel_ganging - output connected.vi"("error in (no error)"=w445, "output enabled"=w443, "Ganged Session In"=w444) -> ("error out"=w446:errorcluster, "Ganged Session Out"=w447:T8)  [unwired: 7 in]
      n152 = call "NIDCPower_channel_ganging - reset.vi"("error in (no error)"=w446, "Ganged Session In"=w447) -> ("error out"=w433:errorcluster, "Ganged Session Out"=w434:T8)  [unwired: 8 in]
      n153 = call "NIDCPower_channel_ganging - close.vi"("error in (no error)"=w433, "Ganged Session In"=w434) -> ("error out"=w421:errorcluster)  [unwired: 9 in]
      n154 = call "Get Channel List.vi"("error in (no error)"=w421, "Slave resource names"=w419, "Master resouce name"=w420) -> ("error out"=w428:errorcluster, "Channel List"=w427:T6[])  [unwired: 7 in]
      n155 = call "NIDCPower_channel_ganging - initialize.vi"("Ganged Config"=w449, "error in (no error)"=w428, "Channel List"=w427) -> ("error out"=w429:errorcluster, "Ganged Session Out"=w430:T8)  [unwired: 7 in]
      n156 = call "NIDCPower_channel_ganging - output enabled.vi"("error in (no error)"=w429, "output enabled"=w426, "Ganged Session In"=w430) -> ("error out"=w424:errorcluster, "Ganged Session Out"=w425:T8)  [unwired: 7 in]
      n157 = call "NIDCPower_channel_ganging - output connected.vi"("error in (no error)"=w424, "output enabled"=w426, "Ganged Session In"=w425) -> ("error out"=w423:errorcluster, "Ganged Session Out"=w422:T8)  [unwired: 7 in]
      n158 = call "NIDCPower_channel_ganging - reset.vi"("error in (no error)"=w423, "Ganged Session In"=w422) -> ("error out"=w432:errorcluster, "Ganged Session Out"=w431:T8)  [unwired: 8 in]
      n159 = call "NIDCPower_channel_ganging - close.vi"("error in (no error)"=w432, "Ganged Session In"=w431) -> ("error out"=w417:errorcluster)  [unwired: 9 in]
      n160 = Bundle By Name(cluster=w418, "Status"=w414, "Status (Load)"=w414) -> (w416:T1)
    }
  }
  "error out" <- w6
  "measurement results" <- w8
  "measure call context out" <- w7
